vi "OP500Z8P_CurrentCompare.vi"(8 "errin":errorcluster, 10 "Consigne":dbl, 11 "ITECH VISA NAME":refnum<visa-resource-name>) -> (0 "errout":errorcluster, 1 "Courant OK ?":bool, 2 "BDU Current (A)":dbl, 3 "Itech Current (A)":dbl format="%.2g", 4 "BMS Current (A)":string)   [LabVIEW 2020]
uses:
  <userlib>/PCAN Basic/Controls/BaudrateEenum.ctl
  <userlib>/PCAN Basic/Controls/Channel.ctl
  VG/VG_Ibms.vi
  <instrlib>/IT6000C/IT6000C.lvlib
  <userlib>/PCAN Basic/PCANBasic.lvlib
panel:
  out "I inst":dbl
  in  "Stop":bool
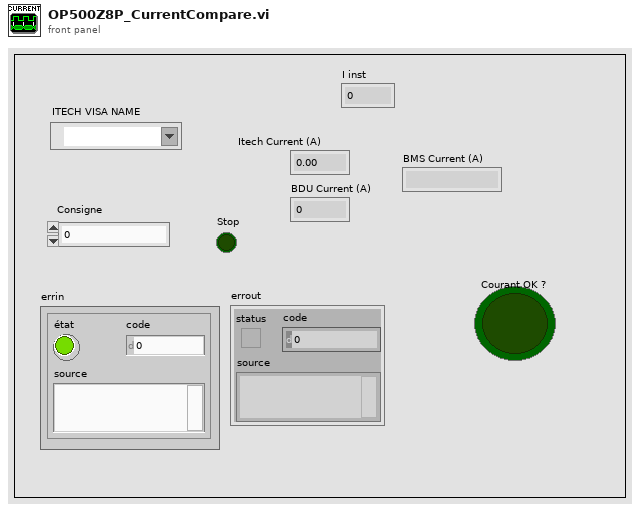
[diagram p1: front panel]
types:
  T1 = typedef "PCANBasic.lvlib/Channel.ctl" = enum16{"PCAN_NONEBUS", "not used1", "not used2", "not used3", "not used4", "not used5", "not used6", "not used7", "not used8", "not used9", "not used10", "not used11", "not used12", "not used13", "not used14", "not used15", "not used16", "not used17", "not used18", "not used19", "not used20", "not used21", "not used22", "not used23", "not used24", "not used25", "not used26", "not used27", "not used28", "not used29", "not used30", "not used31", "not used32", "PCAN_ISABUS1", "PCAN_ISABUS2", "PCAN_ISABUS3", "PCAN_ISABUS4", "PCAN_ISABUS5", "PCAN_ISABUS6", "PCAN_ISABUS7", "PCAN_ISABUS8", "not used41", "not used42", "not used43", "not used44", "not used45", "not used46", "not used47", "not used48", "PCAN_DNGBUS1", "not used50", "not used51", "not used52", "not used53", "not used54", "not used55", "not used56", "not used57", "not used58", "not used59", "not used60", "not used61", "not used62", "not used63", "not used64", "PCAN_PCIBUS1", "PCAN_PCIBUS2", "PCAN_PCIBUS3", "PCAN_PCIBUS4", "PCAN_PCIBUS5", "PCAN_PCIBUS6", "PCAN_PCIBUS7", "PCAN_PCIBUS8", "not used73", "not used74", "not used75", "not used76", "not used77", "not used78", "not used79", "not used80", "PCAN_USBBUS1", "PCAN_USBBUS2", "PCAN_USBBUS3", "PCAN_USBBUS4", "PCAN_USBBUS5", "PCAN_USBBUS6", "PCAN_USBBUS7", "PCAN_USBBUS8", "Not used89", "Not used90", "Not used91", "Not used92", "Not used93", "Not used94", "Not used95", "Not used96", "PCAN_PCCBUS1", "PCAN_PCCBUS2"}
  T2 = typedef "PCANBasic.lvlib/BaudrateEenum.ctl" = enum16{"CAN_Baud_1M", "CAN_Baud_800K", "CAN_BAUD_500K", "CAN_BAUD_250K", "CAN_BAUD_125K", "CAN_BAUD_100K", "CAN_BAUD_95K", "CAN_BAUD_83K", "CAN_BAUD_50K", "CAN_BAUD_47K", "CAN_BAUD_33K", "CAN_BAUD_20K", "CAN_BAUD_10K", "CAN_BAUD_5K", "User Baudrate"}
  T3 = typedef "PCANBasic.lvlib/CAN MSG Cluster.ctl" = cluster{"ID":u32, "MSG type":enum8{"STD", "RTR", "XTD", "XTD RTR", "STATUS"}, "LEN":i8, "DATA":u8[]}
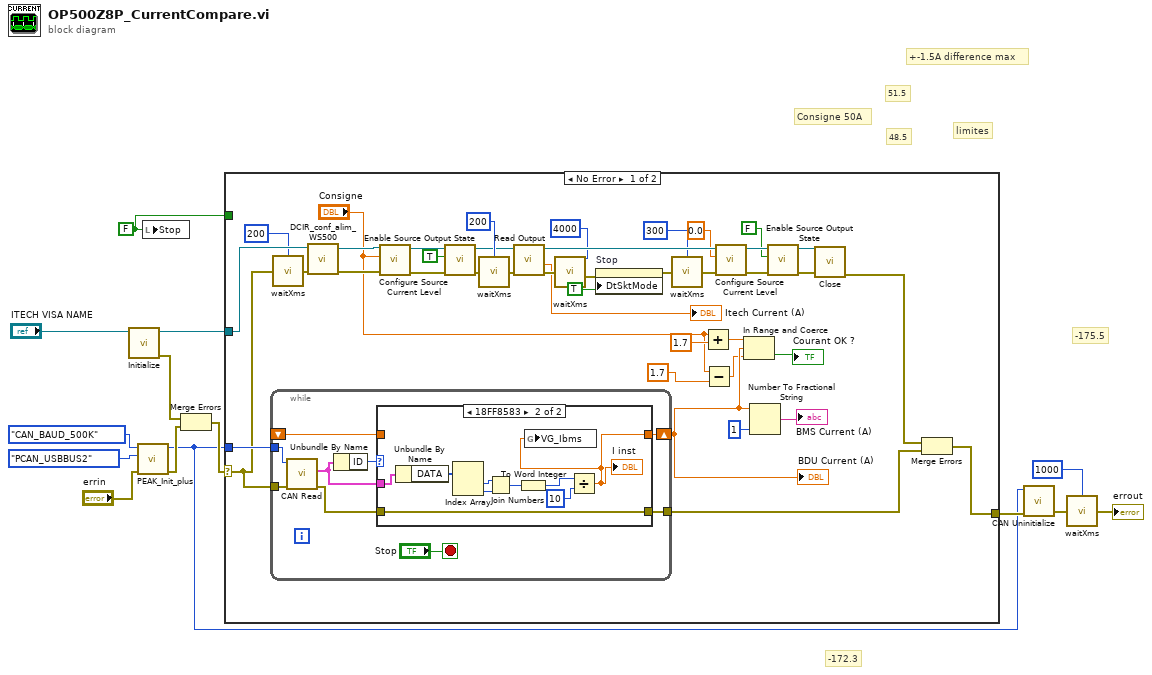
[diagram p0: block diagram]
diagram:
  w1 = FALSE ("Stop")
  # "-175.5"
  # "-172.3"
  # "+-1.5A difference max"
  # "limites"
  # "48.5"
  # "51.5"
  # "Consigne 50A"
  n1 = call <instrlib>:"Initialize.vi"("VISA resource name"="ITECH VISA NAME") -> ("error out"=w9:errorcluster, "VISA resource name out"=w6:refnum<visa-resource-name>)  [unwired: 9 in]
  n2 = call <userlib>:"PEAK_Init_plus.vi"("errin"="errin", "Channel"=Channel."PCAN_USBBUS2", "BTR0BTR1"=BaudrateEenum."CAN_BAUD_500K") -> ("errout"=w8:errorcluster, "Channel out"=w5:T1)  [unwired: 7 in]
  n3 = local write "Stop"(w1) -> ()
  n4 = Merge Errors(w9, w8) -> (w7:errorcluster)
  n5 = case shown="No Error" w7 {
    selector: w7 -> [w22 w76]
    tunnel: w5 -> [w55 _]
    tunnel: [w37 w76] -> w10
    tunnel: w6 -> [w40 _]
    tunnel: w1 -> [_ _]
    frame No Error {
      n6 = while {
        tunnel: w55 -> [w64]
        tunnel: [w59] -> w38
        shift-right: [w61] -> w28
        shift-left: _ -> [w58]
        tunnel: w22 -> [w57]
        stop <- "Stop" stop-if-true
        n7 = call <userlib>:"CAN Read.vi"("error in (no error)"=w57, "Channel"=w64) -> ("error out"=w60:errorcluster, "CAN_Message out"=w62:T3)  [unwired: 5 in, 3 out]
        n8 = Unbundle By Name(w62) -> ("ID"=w63:u32)
        n9 = case shown="18FF8583" w63 {
          tunnel: w62 -> [_ w75]
          tunnel: [w65 w67] -> w61
          tunnel: w60 -> [w66 w73]
          tunnel: [w66 w73] -> w59
          tunnel: w58 -> [w65 _]
          frame 0, Default {
          }
          frame 419399043 {
            n10 = Unbundle By Name(w75) -> ("DATA"=w74:u8[])
            n11 = Index Array(array=w74) -> (element #1=w71:u8, element #2=w72:u8)  [unwired: 2 in]
            n12 = Join Numbers(hi=w71, lo=w72) -> ((hi.lo)=w70:u16)
            n13 = To Word Integer(number=w70) -> (16bit integer=w69:i16)
            n14 = Divide(x=w69, y=i16 10) -> (x/y=w67:dbl)
            "I inst" <- w67
            n15 = global write "VG_Ibms.vi" "VG_Ibms"(w67) -> ()
          }
        }
      }
      "BDU Current (A)" <- w28
      n16 = call <userlib>:"waitXms.vi"("attente (ms)"=u32 200, "errin"=w22) -> ("errout"=w23:errorcluster)  [unwired: 13 in]
      n17 = call "DCIR_conf_alim_WS500.vi"("ErrIN"=w23, "VISAin"=w40) -> ("ErrOUT"=w45:errorcluster, "VisaOUT"=w46:refnum<visa-resource-name>)  [unwired: 8 in]
      n18 = call <instrlib>:"Configure Source Current Level.vi"("error in (no error)"=w45, "Value(0)"="Consigne", "VISA resource name"=w46) -> ("error out"=w47:errorcluster, "VISA resource name out"=w48:refnum<visa-resource-name>)  [unwired: 7 in]
      n19 = call <instrlib>:"Enable Source Output State.vi"("error in (no error)"=w47, "Enable(True)"=TRUE, "VISA resource name"=w48) -> ("error out"=w36:errorcluster, "VISA resource name out"=w33:refnum<visa-resource-name>)  [unwired: 7 in]
      n20 = call <userlib>:"waitXms.vi"("attente (ms)"=u32 200, "errin"=w36) -> ("errout"=w35:errorcluster)  [unwired: 13 in]
      n21 = call <instrlib>:"Read Output.vi"("error in (no error)"=w35, "VISA resource name"=w33) -> ("error out"=w54:errorcluster, "Actual Current Level (A)"=→"Itech Current (A)":dbl, "VISA resource name out"=w49:refnum<visa-resource-name>)  [unwired: 6 in, 1 out]
      n22 = call <userlib>:"waitXms.vi"("attente (ms)"=u32 4000, "errin"=w54) -> ("errout"=w20:errorcluster)  [unwired: 13 in]
      n23 = property on="Stop" class="Bool (strict)"(error in=w20, "DtSktMode"=TRUE ("Stop")) -> (error out=w17:errorcluster)  [unwired: 1 in, 1 out]
      n24 = call <userlib>:"waitXms.vi"("attente (ms)"=u32 300, "errin"=w17) -> ("errout"=w16:errorcluster)  [unwired: 13 in]
      n25 = Add(x="Consigne", y=1.7) -> (x+y=w29:dbl)
      n26 = Subtract(x="Consigne", y=1.7) -> (x-y=w25:dbl)
      n27 = call <instrlib>:"Configure Source Current Level.vi"("error in (no error)"=w16, "Value(0)"=0.0, "VISA resource name"=w49) -> ("error out"=w51:errorcluster, "VISA resource name out"=w50:refnum<visa-resource-name>)  [unwired: 7 in]
      n28 = In Range and Coerce(upper limit=w29, x=w28, lower limit=w25) -> (In Range?=→"Courant OK ?":bool)  [unwired: 1 out]
      n29 = Number To Fractional String(number=w28, precision (6)=i16 1) -> (F-format string=→"BMS Current (A)":string)  [unwired: 2 in]
      n30 = call <instrlib>:"Enable Source Output State.vi"("error in (no error)"=w51, "Enable(True)"=FALSE, "VISA resource name"=w50) -> ("error out"=w52:errorcluster, "VISA resource name out"=w53:refnum<visa-resource-name>)  [unwired: 7 in]
      n31 = call <instrlib>:"Close.vi"("error in (no error)"=w52, "VISA resource name"=w53) -> ("error out"=w39:errorcluster)  [unwired: 9 in]
      n32 = Merge Errors(w39, w38) -> (w37:errorcluster)
    }
    frame Error {
    }
  }
  n33 = call <userlib>:"CAN Uninitialize.vi"("error in (no error)"=w10, "Channel"=w5) -> ("error out"=w4:errorcluster)  [unwired: 7 in, 2 out]
  n34 = call <userlib>:"waitXms.vi"("attente (ms)"=u32 1000, "errin"=w4) -> ("errout"=→"errout":errorcluster)  [unwired: 13 in]
